vi "simple_examples.vi"() -> ()   [LabVIEW 2018, in "LV-0mq-Julia_roundtrip-lib.lvlib"]
uses:
  LV-0mq-Julia_roundtrip-lib.lvlib
  Server or client state.ctl
  detailed error info.ctl
  StackFrame.ctl
  simple examples functions.ctl
  Commands.ctl
  edf81fa3-46bf-427f-9605-85b461656974.vi
  d2cb43a9-9305-42fb-ad58-bce983510195.vi
  9182218e-1e17-4e73-8c4b-7de0f475a335.vi
  35a44a82-786b-41ea-be73-9a4468e4df9d.vi
  edf81fa3-46bf-427f-9605-85b461656974.vi/dd2a08ad-0639-467b-9435-389f4bd48a85.vi
  d2cb43a9-9305-42fb-ad58-bce983510195.vi/e28c4e1c-617d-4a26-8291-f58a5accd33d.vi
  d2cb43a9-9305-42fb-ad58-bce983510195.vi/697b26af-9cff-4296-98ec-fa9d12ca8fdc.vi
  d2cb43a9-9305-42fb-ad58-bce983510195.vi/17159f77-75f5-4b7b-8d47-844af2eb1bcd.vi
  9182218e-1e17-4e73-8c4b-7de0f475a335.vi/6b7feeb5-19de-417f-bcbc-aec3b1e8345f.vi
  9182218e-1e17-4e73-8c4b-7de0f475a335.vi/7970c5bc-6f8c-498d-9eee-822ea5f26e23.vi
  9182218e-1e17-4e73-8c4b-7de0f475a335.vi/2f2cc08c-6f15-46a0-b24a-2c0737e5dd5e.vi
  35a44a82-786b-41ea-be73-9a4468e4df9d.vi/edd291af-888e-4547-8763-33a9db2b2a61.vi
  35a44a82-786b-41ea-be73-9a4468e4df9d.vi/9c0ac3f0-dad9-4795-8f5f-702d875dafaa.vi
  edf81fa3-46bf-427f-9605-85b461656974.vi/dd2a08ad-0639-467b-9435-389f4bd48a85.vi/1040e0bc-00ab-48b1-9004-b2897991f2c6.vi
  35a44a82-786b-41ea-be73-9a4468e4df9d.vi/edd291af-888e-4547-8763-33a9db2b2a61.vi/c75629c6-22a1-4cf2-848a-1de687213dd2.vi
  35a44a82-786b-41ea-be73-9a4468e4df9d.vi/edd291af-888e-4547-8763-33a9db2b2a61.vi/58d0dd4f-d013-483e-a73a-a72c22b2f5d6.vi
  edf81fa3-46bf-427f-9605-85b461656974.vi/dd2a08ad-0639-467b-9435-389f4bd48a85.vi/1040e0bc-00ab-48b1-9004-b2897991f2c6.vi/e9506487-c1a2-4aa8-b83c-f353e91e5b82.vi
  35a44a82-786b-41ea-be73-9a4468e4df9d.vi/edd291af-888e-4547-8763-33a9db2b2a61.vi/c75629c6-22a1-4cf2-848a-1de687213dd2.vi/f86c6b3b-20ab-4607-a249-4edff951d1c3.vi
  jl-scripts path.vi
  check ID validity.vi
  bindata_descr to JSON.vi
  check cluster field names.vi
  concat JSON.vi
  <vilib>/Utility/error.llb/Error Cluster From Error Code.vi
  <vilib>/measure/NI_MABase.lvlib
panel:
  out "ZMQ timeout":bool
  out "Julia script file path":path
  out "temporary script path":path
  out "Jl Server state":T1
  in  "execution control pages":enum32{"Start", "go - test"}(tab)
  in  "go":bool caption="go (Julia Server started externally)"
  in  "Start with Julia":bool caption="Start Julia Server and go"
  in  "ZMQ endpoint":string="tcp://127.0.0.1:5555"
  in  "p":dbl=1.0
  in  "fn":T2 caption="select function at Server" items=["arr_amplitude", "arr_length", "arr_mean", "arr_median", "arr_rms", "vec_amplify", "vec_attenuate", "vec_power"]
  in  "trim_at_begin":dbl
  in  "trim_at_end":dbl
  in  "Group":T3(tab)
  out "Server response":dbl
  out "data received plot":dbl[](graph)
  out "data received":dbl[](array[numeric]) format="%.3f"
  out "RMS":dbl
  out "detailed error info":T4
  out "current error":errorcluster
  out "final error":errorcluster
  out "short err code":u8
  in  "tones":T6(array[cluster])=[{"frequency"=10.0, "amplitude"=1.0, "phase"=0.0}, {"frequency"=20.0, "amplitude"=0.1, "phase"=0.0}] {"phase" format="%.2p"; "amplitude" format="%0.2p"; "frequency" format="%0.2p"}
  in  "noise (rms)":dbl=0.1 format="%.2p"
  in  "offset":dbl format="%.2p"
  in  "sampling info":cluster{"Fs":dbl, "#s":dbl}={"Fs"=1000.0, "#s"=1000.0} {"Fs" format="%.2p"}
  in  "next":bool
  out "data sent to server":dbl[](graph)
  out "data sent":dbl[](array[numeric]) format="%.3f"
  out "function name":string
  in  "stop this VI only":bool
  in  "stop both this VI and Julia Server":bool
  # "tcp://127.0.0.1:5555 \nfor local Julia Server\n\nUsed only if Julia Server is not being started by this VI"
  # "generate sample array"
  # "function and parameter"
  # "enter a negative or a large positive value to cause an exception"
  # "data returned by server"
  # "data sent to server"
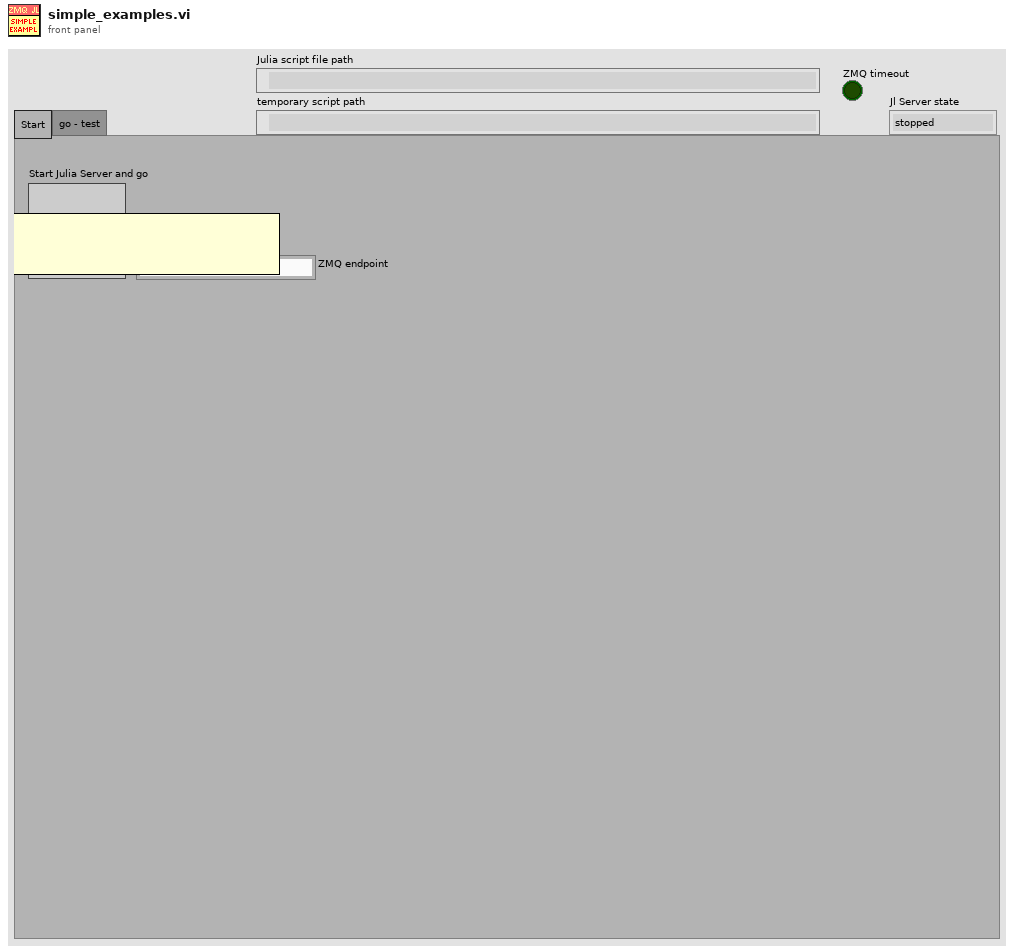
[diagram p1: front panel]
types:
  T1 = typedef "LV-0mq-Julia_roundtrip-lib.lvlib/Server or client state.ctl" = enum16{"stopped", "running", "unknown"}
  T2 = typedef "LV-0mq-Julia_roundtrip-lib.lvlib/simple examples functions.ctl" = u16
  T3 = enum32{"fns returning scalar", "fns returning vector", "error"}
  T4 = typedef "LV-0mq-Julia_roundtrip-lib.lvlib/detailed error info.ctl" = cluster{"exception_or_info":string, "trace":T5[]}
  T5 = typedef "LV-0mq-Julia_roundtrip-lib.lvlib/StackFrame.ctl" = cluster{"frame_summary":string, "func":string, "linfo":string, "file":string, "line":i32, "pointer":u64, "from_c":bool, "inlined":bool}
  T6 = cluster{"frequency":dbl, "amplitude":dbl, "phase":dbl}[]
  T7 = typedef "LV-0mq-Julia_roundtrip-lib.lvlib/Commands.ctl" = enum16{"Start Jl-server & Init LV-client", "Send request & Get response ", "Stop Jl-server & Cleanup LV-client", "Cleanup LV-client", "Start Jl-server", "Stop Jl-server", "Init LV-Client", "Cleanup LV-Client", "(not allowed)", "Set LV Client state", "Set Jl Server state", "set ZMQ timeout", "read ZMQ timeout", "read-out state"}
  T8 = enum8{"Enabled", "Disabled", "Disabled and Grayed Out"}
  T9 = typedef "LV-0mq-Julia_roundtrip-lib.lvlib/Bindata&description.ctl" = cluster{"bindata_descr":T10[], "bindata":u8[]}
  T10 = typedef "LV-0mq-Julia_roundtrip-lib.lvlib/Bindata description.ctl" = cluster{"nofbytes":i32, "numtype":string, "start":i32, "arrdims":i32[], "kwarg_name":string, "category":string}
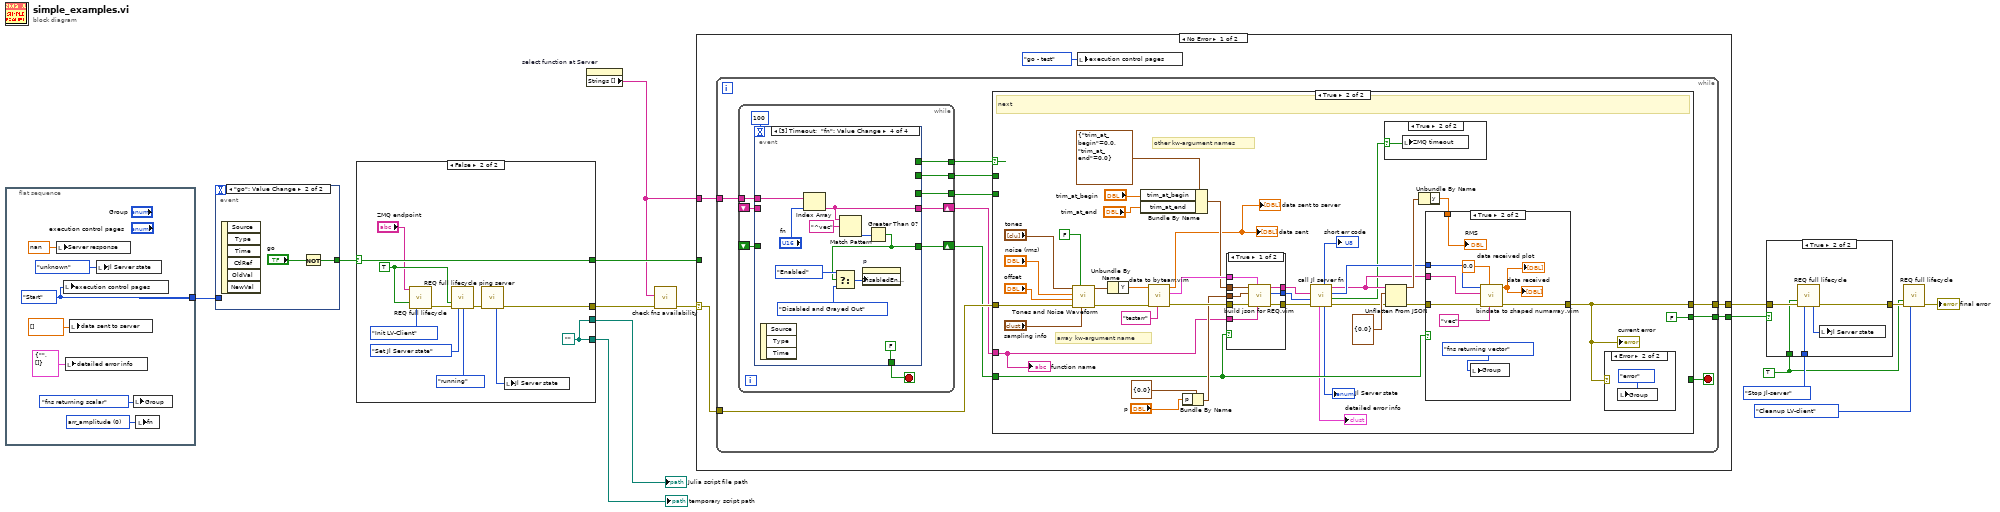
[diagram p0: block diagram]
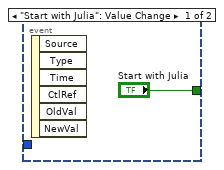
[diagram p2: hidden frame]
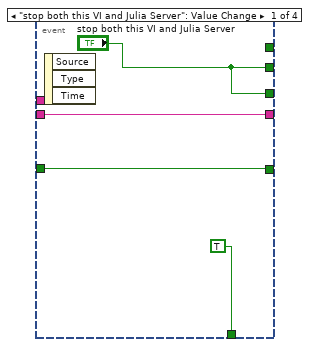
[diagram p3: hidden frame]
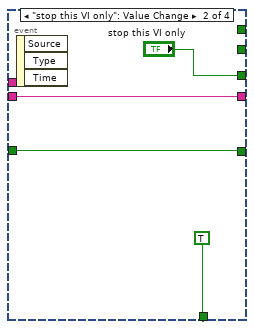
[diagram p4: hidden frame]
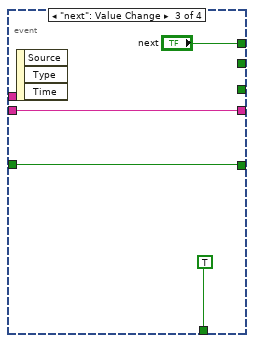
[diagram p5: hidden frame]
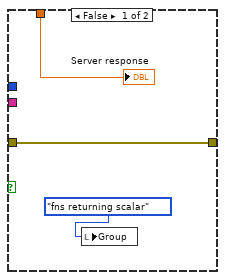
[diagram p8: hidden frame]
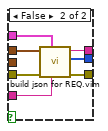
[diagram p9: hidden frame]
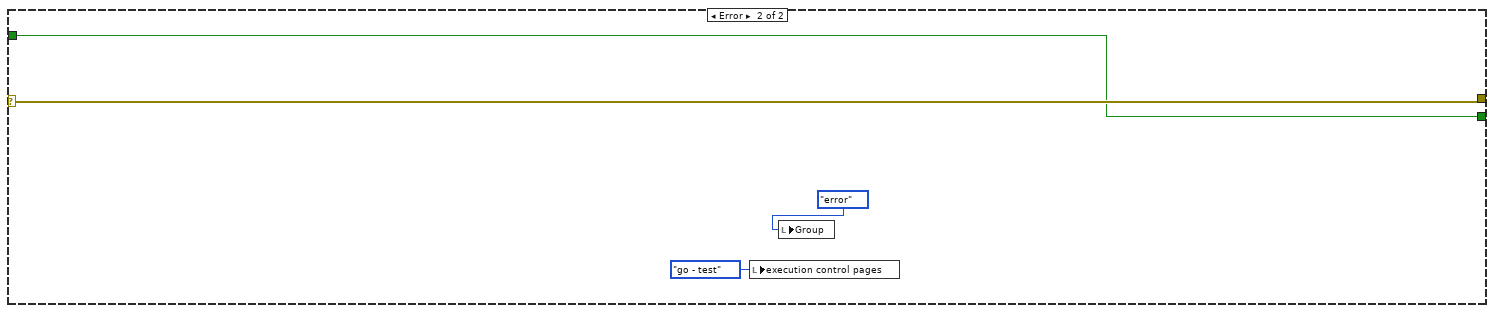
[diagram p11: hidden frame]
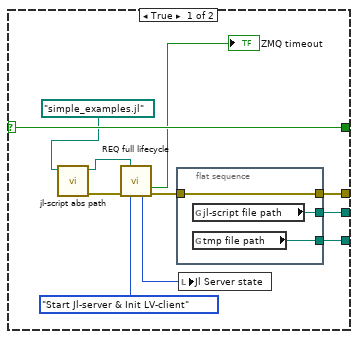
[diagram p12: hidden frame]
diagram:
  w10 = TRUE ("Force command")
  n1 = flat-sequence {
    tunnel: [w22] -> w6
    frame #0 {
      w16 = T2 0 items=["arr_amplitude", "arr_length", "arr_mean", "arr_median", "arr_rms", "vec_amplify", "vec_attenuate", "vec_power"] ("fn")
      w22 = enum32{"Start", "go - test", "finish"}."Start" ("execution control pages")
      n2 = local write "Server response"(nan ("Server response")) -> ()
      n3 = local write "execution control pages"(w22) -> ()
      n4 = local write "detailed error info"(T4 {"exception_or_info"="", "trace"=[]} ("detailed error info")) -> ()
      n5 = local write "data sent to server"(dbl[] []) -> ()
      n6 = local write "Jl Server state"(Server_or_client_state."unknown" ("Jl Server state out")) -> ()
      n7 = local write "Group"(T3."fns returning scalar" ("Group")) -> ()
      n8 = local write "fn"(w16) -> ()
    }
  }
  n9 = event shown="[1] \"go\": Value Change" {
    selector: _ -> [_ _]
    dyn-events: _ -> [_ _]
    timeout: _ -> [_ _]
    tunnel: ["Start with Julia" w24] -> w8
    tunnel: w6 -> [_ _]
    event "Start with Julia": Value Change {
      n10 = event-data() -> ()  [unwired: 1 in, 6 out]
    }
    event "go": Value Change {
      n11 = event-data() -> ()  [unwired: 1 in, 6 out]
      n12 = Not(x="go") -> (.not. x?=w24:bool)
    }
  }
  n13 = case shown="False" w8 {
    selector: w8 -> [w35 w46]
    tunnel: [w32 w42] -> w5
    tunnel: [w35 w46] -> w7
    tunnel: [w31 w41] -> w1
    tunnel: [w30 w41] -> w2
    frame True {
      n14 = call "jl-script abs path.vi"("Julia user functions script"=path "simple_examples.jl") -> ("error out"=w28:errorcluster, "script abs path"=w29:path)  [unwired: 9 in]
      n15 = call "REQ full lifecycle.vi"("Julia user functions script"=w29, "error in"=w28, "command"=Commands."Start Jl-server & Init LV-client") -> ("timeout?"=→"ZMQ timeout":bool, "Jl Server state out"=w34:T1, "error out"=w33:errorcluster)  [unwired: 6 in, 4 out]
      n16 = flat-sequence {
        tunnel: [w39] -> w32
        tunnel: w33 -> [w39]
        tunnel: [w38] -> w31
        tunnel: [w37] -> w30
        frame #0 {
          n17 = global read "jl-scripts path.vi" "jl-script file path"() -> (w38:path)
          n18 = global read "jl-scripts path.vi" "tmp file path"() -> (w37:path)
        }
      }
      n19 = local write "Jl Server state"(w34) -> ()
    }
    frame False {
      w41 = path ""
      w48 = TRUE ("Force command")
      n20 = call "REQ full lifecycle.vi"("ZMQ endpoint"="ZMQ endpoint", "Force command"=w48, "command"=Commands."Init LV-Client") -> ("error out"=w45:errorcluster)  [unwired: 6 in, 6 out]
      n21 = call "REQ full lifecycle.vi"("Force command"=w48, "error in"=w45, "command"=Commands."Set Jl Server state", "Jl Server state in"=Server_or_client_state."running") -> ("error out"=w44:errorcluster)  [unwired: 5 in, 6 out]
      n22 = call "ping server.vi"("error in"=w44) -> ("error out"=w42:errorcluster, "Jl Server state out"=w43:T1)  [unwired: 6 in, 3 out]
      n23 = local write "Jl Server state"(w43) -> ()
    }
  }
  "temporary script path" <- w2
  "Julia script file path" <- w1
  n24 = property on="select function at Server" class="Ring (strict)"() -> ("Strings []"=w3:string[])  [unwired: 2 in, 2 out]
  n25 = call "check fns availability.vi"("error in (no error)"=w5, "fns list is"=w3) -> ("error out"=w4:errorcluster)  [unwired: 3 in, 6 out]
  n26 = case shown="No Error" w4 {
    selector: w4 -> [w54 w171]
    tunnel: [w55 w171] -> w15
    tunnel: [w53 w170] -> w9
    tunnel: w3 -> [w52 _]
    tunnel: w7 -> [_ w170]
    frame No Error {
      n27 = while {
        tunnel: w54 -> [w64]
        tunnel: [w65] -> w55
        tunnel: [w61] -> w53
        tunnel: w52 -> [w59]
        stop <- w62 stop-if-true
        n28 = while {
          tunnel: [w75] -> w63
          tunnel: [w74] -> w60
          tunnel: w59 -> [w71]
          shift-right: [w70] -> w58
          shift-left: _ -> [w67]
          shift-right: [w69] -> w57
          shift-left: _ -> [w68]
          tunnel: [w66] -> w56
          stop <- w73 stop-if-true
          n29 = event shown="[3] Timeout;  \"fn\": Value Change" {
            selector: _ -> [_ _ _ _]
            dyn-events: _ -> [_ _ _ _]
            timeout: 100 -> [_ _ _ _]
            tunnel: ["stop both this VI and Julia Server" _ _ _] -> w74
            tunnel: [_ _ "next" _] -> w75
            tunnel: [TRUE TRUE TRUE FALSE] -> w73
            tunnel: w71 -> [_ _ _ w91]
            tunnel: [w77 w81 w85 w90] -> w70
            tunnel: [w78 w82 w84 w89] -> w69
            tunnel: w68 -> [w78 w82 w84 _]
            tunnel: w67 -> [w77 w81 w85 _]
            tunnel: ["stop both this VI and Julia Server" "stop this VI only" _ _] -> w66
            event "stop both this VI and Julia Server": Value Change {
              n30 = event-data() -> ()  [unwired: 1 in, 3 out]
            }
            event "stop this VI only": Value Change {
              n31 = event-data() -> ()  [unwired: 1 in, 3 out]
            }
            event "next": Value Change {
              n32 = event-data() -> ()  [unwired: 1 in, 3 out]
            }
            event Timeout; Value Change {
              n33 = event-data() -> ()  [unwired: 1 in, 3 out]
              n34 = Index Array(array=w91, index="fn") -> (element=w89:string)
              n35 = Match Pattern(string=w89, regular expression="^vec") -> (offset past match=w95:i32)  [unwired: 1 in, 3 out]
              n36 = Greater Than 0?(x=w95) -> (x > 0?=w90:bool)
              n37 = Select(t=T8."Enabled" ("Disabled"), s=w90, f=T8."Disabled and Grayed Out" ("Disabled")) -> (s? t:f=w97:T8)
              n38 = property on="p" class="DigNum (strict)"("DisabledEnum"=w97) -> ()  [unwired: 2 in, 2 out]
            }
          }
        }
        n39 = case shown="True" w63 {
          tunnel: [w100 w114] -> w65
          tunnel: w64 -> [w100 w121]
          tunnel: [w99 w119] -> w62
          tunnel: w56 -> [w99 _]
          tunnel: [w98 w119] -> w61
          tunnel: w60 -> [w98 _]
          tunnel: w58 -> [_ w112]
          tunnel: w57 -> [_ w111]
          frame False {
            # "stop"
          }
          frame True {
            w119 = FALSE ("stop this VI only")
            # "other kw-argument names"
            # "array kw-argument name"
            # "next"
            n40 = call <vilib>:"Tones and Noise Waveform.vi"("sampling info"="sampling info", "reset signal"=FALSE, "error in (no error)"=w121, "offset"="offset", "noise (rms)"="noise (rms)", "tones"="tones") -> ("error out"=w122:errorcluster, "signal out"=w128:waveform(dbl))  [unwired: 4 in]
            n41 = Unbundle By Name(w128) -> ("Y"=w123:dbl[])
            n42 = Bundle By Name(cluster=cluster{"trim_at_begin":dbl, "trim_at_end":dbl} {"trim_at_begin"=0.0, "trim_at_end"=0.0}, "trim_at_begin"="trim_at_begin", "trim_at_end"="trim_at_end") -> (w132:cluster{"trim_at_begin":dbl, "trim_at_end":dbl})
            n43 = call "data to bytearr.vim"("kwarg_name"="testarr", "error in (no error)"=w122, "data in"=w123) -> ("error out"=w135:errorcluster, "Bindata & descr out"=w136:T9, "flattened data out"=→"data sent" →"data sent to server":dbl[])  [unwired: 6 in]
            n44 = Bundle By Name(cluster=cluster{"p":dbl} {"p"=0.0}, "p"="p") -> (w118:cluster{"p":dbl})
            n45 = case shown="True" w112 {
              tunnel: [w159 w166] -> w108
              tunnel: [w158 w165] -> w110
              tunnel: [w157 w164] -> w109
              tunnel: w136 -> [w156 w163]
              tunnel: w135 -> [w155 w162]
              tunnel: w132 -> [w154 w161]
              tunnel: w111 -> [w153 w160]
              tunnel: w118 -> [w152 _]
              frame True {
                n46 = call "build json for REQ.vim"("fun2call"=w153, "Bindata & descr in"=w156, "error in (no error)"=w155, "Arguments 2"=w152, "Arguments 1"=w154) -> ("error out"=w159:errorcluster, "bindata out"=w157:u8[], "JSON string out"=w158:string)  [unwired: 4 in]
              }
              frame False {
                n47 = call "build json for REQ.vim"("fun2call"=w160, "Bindata & descr in"=w163, "error in (no error)"=w162, "Arguments 1"=w161) -> ("error out"=w166:errorcluster, "bindata out"=w164:u8[], "JSON string out"=w165:string)  [unwired: 5 in]
              }
            }
            n48 = call "call Jl server fn.vi"("error in (no error)"=w108, "binary data in"=w109, "JSON string in"=w110) -> ("error out"=w102:errorcluster, "timeout?"=w101:bool, "binary data received"=w105:u8[], "JSON received"=w104:string, "Jl Server state out"=→"Jl Server state":T1, "return code"=→"short err code":u8, "detailed error info"=→"detailed error info":T4)  [unwired: 2 in]
            n49 = case shown="True" w101 {
              selector: w101 -> [_ w139]
              frame False {
              }
              frame True {
                n50 = local write "ZMQ timeout"(w139) -> ()
              }
            }
            n51 = Unflatten From JSON(JSON string=w104, type and defaults=cluster{"y":dbl} {"y"=0.0} ("parsed response"), error in (no error)=w102) -> (value=w137:cluster{"y":dbl}, error out=w115:errorcluster)  [unwired: 4 in]
            n52 = Unbundle By Name(w137) -> ("y"=w113:dbl)
            n53 = case shown="True" w112 {
              tunnel: w115 -> [w142 w150]
              tunnel: [w142 w149] -> w114
              tunnel: w105 -> [_ w148]
              tunnel: w104 -> [_ w147]
              tunnel: w113 -> [w140 w144]
              frame False {
                n54 = local write "Group"(T3."fns returning scalar" ("Group")) -> ()
                "Server response" <- w140
              }
              frame True {
                n55 = local write "Group"(T3."fns returning vector" ("Group")) -> ()
                n56 = call "bindata to shaped numarray.vim"("kwarg_name"="vec", "data type"=0.0, "error in (no error)"=w150, "bindata_descr"=w147, "binary data"=w148) -> ("error out"=w149:errorcluster, "numarray 1D"=→"data received plot" →"data received":dbl[])  [unwired: 3 in, 2 out]
                "RMS" <- w144
              }
            }
            "current error" <- w114
            n57 = case shown="Error" w114 {
              frame No Error {
              }
              frame Error {
                n58 = local write "Group"(T3."error" ("Group")) -> ()
              }
            }
            "function name" <- w111
          }
        }
      }
      n59 = local write "execution control pages"(enum32{"Start", "go - test", "finish"}."go - test" ("execution control pages")) -> ()
    }
    frame Error {
      n60 = local write "execution control pages"(enum32{"Start", "go - test", "finish"}."go - test" ("execution control pages")) -> ()
      n61 = local write "Group"(T3."error" ("Group")) -> ()
    }
  }
  n62 = case shown="True" w9 {
    tunnel: w15 -> [w172 w177]
    tunnel: Commands."Stop Jl-server" ("command") -> [_ w176]
    tunnel: [w172 w175] -> w13
    tunnel: w10 -> [_ w174]
    frame False {
    }
    frame True {
      n63 = call "REQ full lifecycle.vi"("Force command"=w174, "error in"=w177, "command"=w176) -> ("Jl Server state out"=w173:T1, "error out"=w175:errorcluster)  [unwired: 6 in, 5 out]
      n64 = local write "Jl Server state"(w173) -> ()
    }
  }
  n65 = call "REQ full lifecycle.vi"("Force command"=w10, "error in"=w13, "command"=Commands."Cleanup LV-client") -> ("error out"=→"final error":errorcluster)  [unwired: 6 in, 6 out]
